vi "global_vision.vi"() -> ()   [LabVIEW 2019]
uses:
  <vilib>/userDefined/High Color/IMAQdx.ctl
panel:
  in  "Global_camera":T2={"ROI-clamp"={"Global Rectangle"=[], "Contours"=[]}, "Clamp Settings"={"Contrast"=0, "Filter width"=0, "Steepness"=0, "Subsampling Ratio"=0, "Show Search Area"=FALSE, "Show Search Lines"=FALSE, "Show Edges Found"=FALSE, "Show Result"=FALSE}, "Angle deg"=0.0, "Image Size"={"x"=0, "y"=0}, "x-center"=0.0, "start_pt-l-out"=[], "start_pt-r-out"=[], "weight-ver-l"=0.0, "weight-ver-r"=0.0, "weight_hor"=0.0, "Replace Value"=0.0, "Threshold Range"={"Lower value"=0.0, "Upper value"=0.0}, "camera cfg"={"Port"="cam2", "Camera file"=path "C:/AGV/Config/camera/C920.icd"}} {"Threshold Range"."Lower value" format="%#_3f"; "Threshold Range"."Upper value" format="%#_3g"}
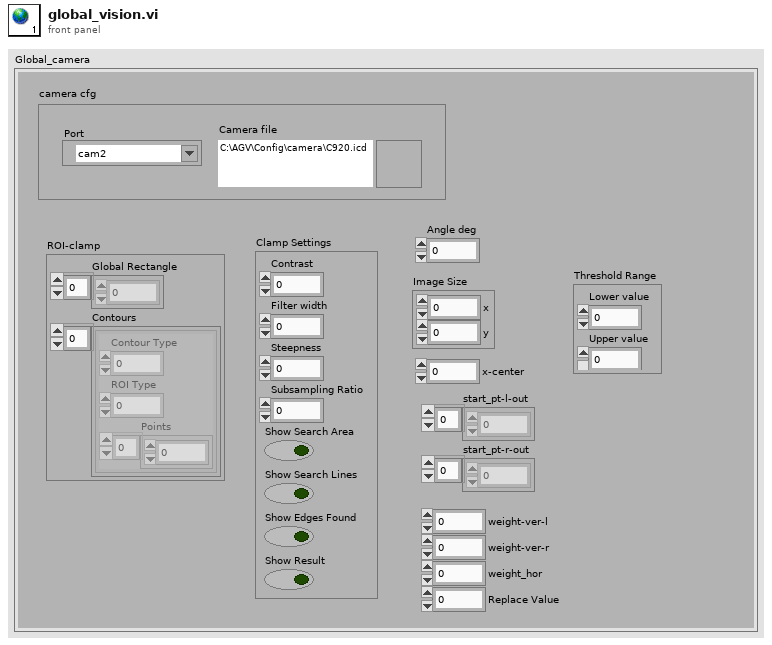
[diagram p1: front panel]
types:
  T1 = typedef "IMAQdx.ctl" = refnum<k21>
  T2 = cluster{"ROI-clamp":cluster{"Global Rectangle":i32[], "Contours":cluster{"Contour Type":u32, "ROI Type":u32, "Points":i32[]}[]}, "Clamp Settings":cluster{"Contrast":i32, "Filter width":i32, "Steepness":i32, "Subsampling Ratio":u32, "Show Search Area":bool, "Show Search Lines":bool, "Show Edges Found":bool, "Show Result":bool}, "Angle deg":sgl, "Image Size":cluster{"x":i32, "y":i32}, "x-center":dbl, "start_pt-l-out":i32[], "start_pt-r-out":i32[], "weight-ver-l":dbl, "weight-ver-r":dbl, "weight_hor":dbl, "Replace Value":sgl, "Threshold Range":cluster{"Lower value":sgl, "Upper value":sgl}, "camera cfg":cluster{"Port":T1, "Camera file":path}}
diagram:
